vi "littleVI_1_DesString.vi"(9 "input_Length":string, 10 "input_AWG":string, 11 "input_sampleDes":string) -> (2 "PNDes":string, 3 "SampleDes":string)   [LabVIEW 2011]
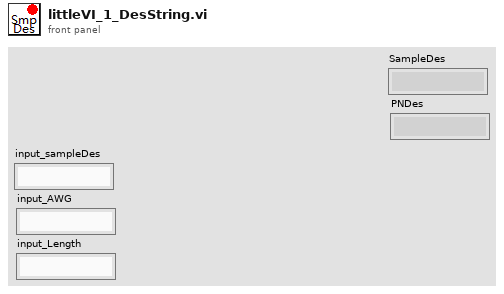
[diagram p1: front panel]
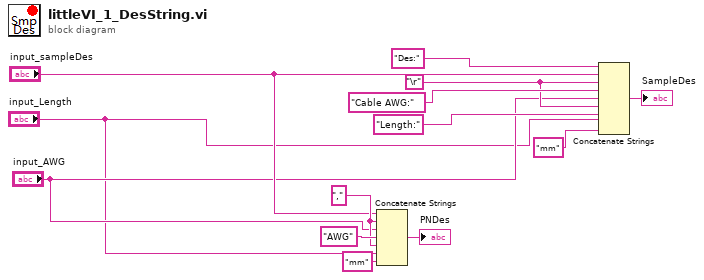
[diagram p0: block diagram]
diagram:
  w7 = "," ("字符串")
  w11 = "\r"
  n1 = Concatenate Strings("input_sampleDes", w7, "input_AWG", "AWG" ("字符串"), w7, "input_Length", "mm" ("字符串")) -> (→"PNDes":string)
  n2 = Concatenate Strings("Des:" ("字符串"), "input_sampleDes", w11, "Cable AWG:" ("字符串"), "input_AWG", w11, "Length:" ("字符串"), "input_Length", "mm" ("字符串")) -> (→"SampleDes":string)
